vi "Get Level.vi"(8 "error in":errorcluster, 11 "Handler in":refnum<class "Handler.lvclass">) -> (0 "error out":errorcluster, 2 "Level":T1, 3 "Handler out":refnum<class "Handler.lvclass">)   [LabVIEW 2016, in "hse-logger.lvlib" / "Handler.lvclass"]
doc: "Returns the log-level of the handler."
uses:
  Handler.lvclass
  LogLevel.ctl
  Handler.lvclass/Handler.ctl
  hse-logger.lvlib
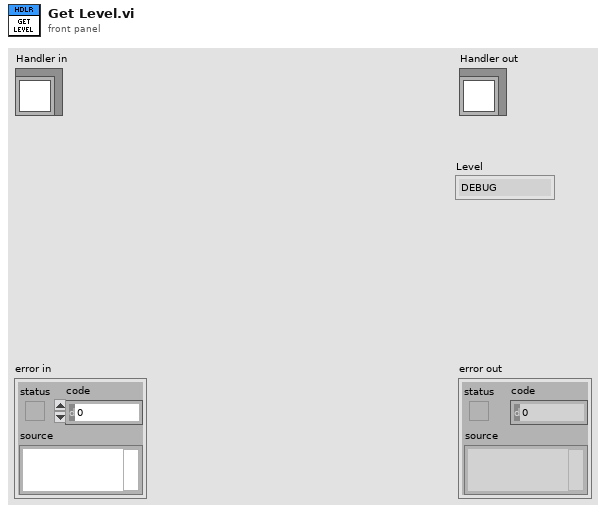
[diagram p1: front panel]
types:
  T1 = typedef "hse-logger.lvlib/LogLevel.ctl" = enum16{"DEBUG", "INFO", "WARNING", "ERROR", "CRITICAL"}
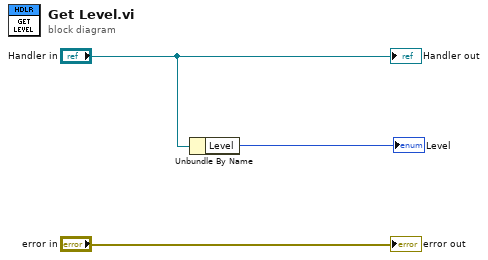
[diagram p0: block diagram]
diagram:
  n1 = Unbundle By Name("Handler in") -> ("Level"=→"Level":T1)
  "error out" <- "error in"
  "Handler out" <- "Handler in"
